vi "ex1.vi"() -> ()   [LabVIEW 2015]
panel:
  in  "stop":bool
  out "Thermometer":dbl(slide) scale=0.0..100.0
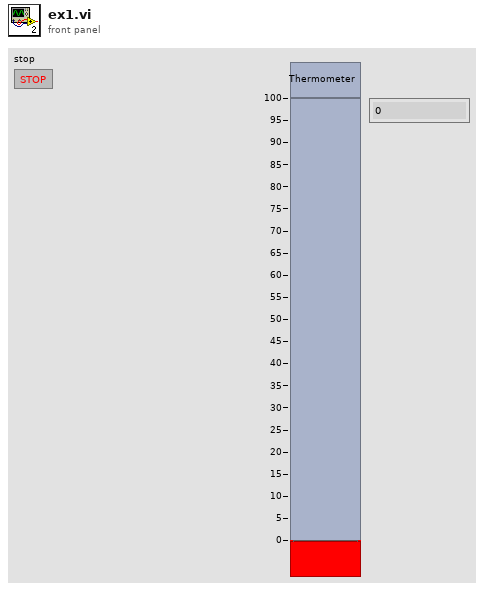
[diagram p1: front panel]
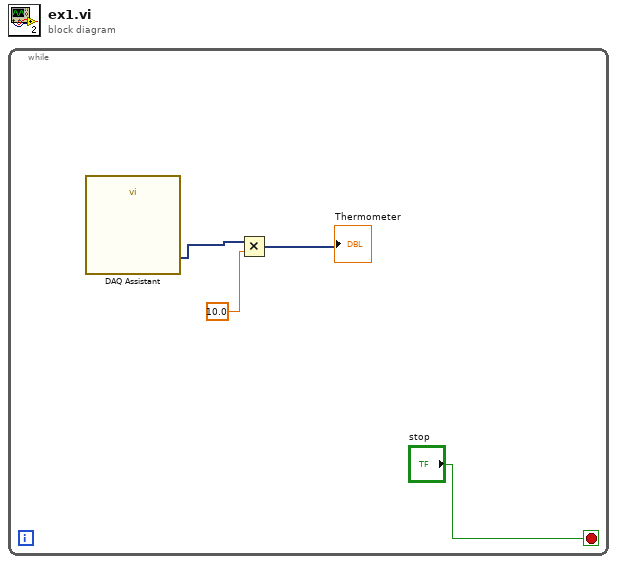
[diagram p0: block diagram]
diagram:
  n1 = while {
    stop <- "stop" stop-if-true
    n2 = call "DAQ Assistant"() -> ("data"=w1:dynamicdata)  [unwired: 16 in, 3 out]
    n3 = Multiply(x=w1, y=10.0) -> (x*y=→"Thermometer":dynamicdata)
  }
